vi "subVI_Mono2Go2Posv2.vi"(0 "Mono2 Motor Pos":refnum<vi>, 1 "Mono2 Wavelength (nm)":refnum<vi>, 2 "HR mode":u16(ring)=3 caption="Which HR?" items=["Excitation"=1, "Detection"=2], 3 "Postion (Unit)":dbl, 4 "ESP300 COM Port":refnum<visa-resource-name>="COM4" caption="COM Port") -> (5 "VISA resource name out":refnum<visa-resource-name>, 6 "error out":errorcluster)   [LabVIEW 2019]
panel:
  in  "Mono2 Wavelength (nm)":dbl=300.0 caption="Wavelength (nm)" min=300.0 max=1000.0 step=0.1
  in  "ESP300 Error":errorcluster
  in  "Mono2 Motor Pos":dbl caption="Motor Pos"
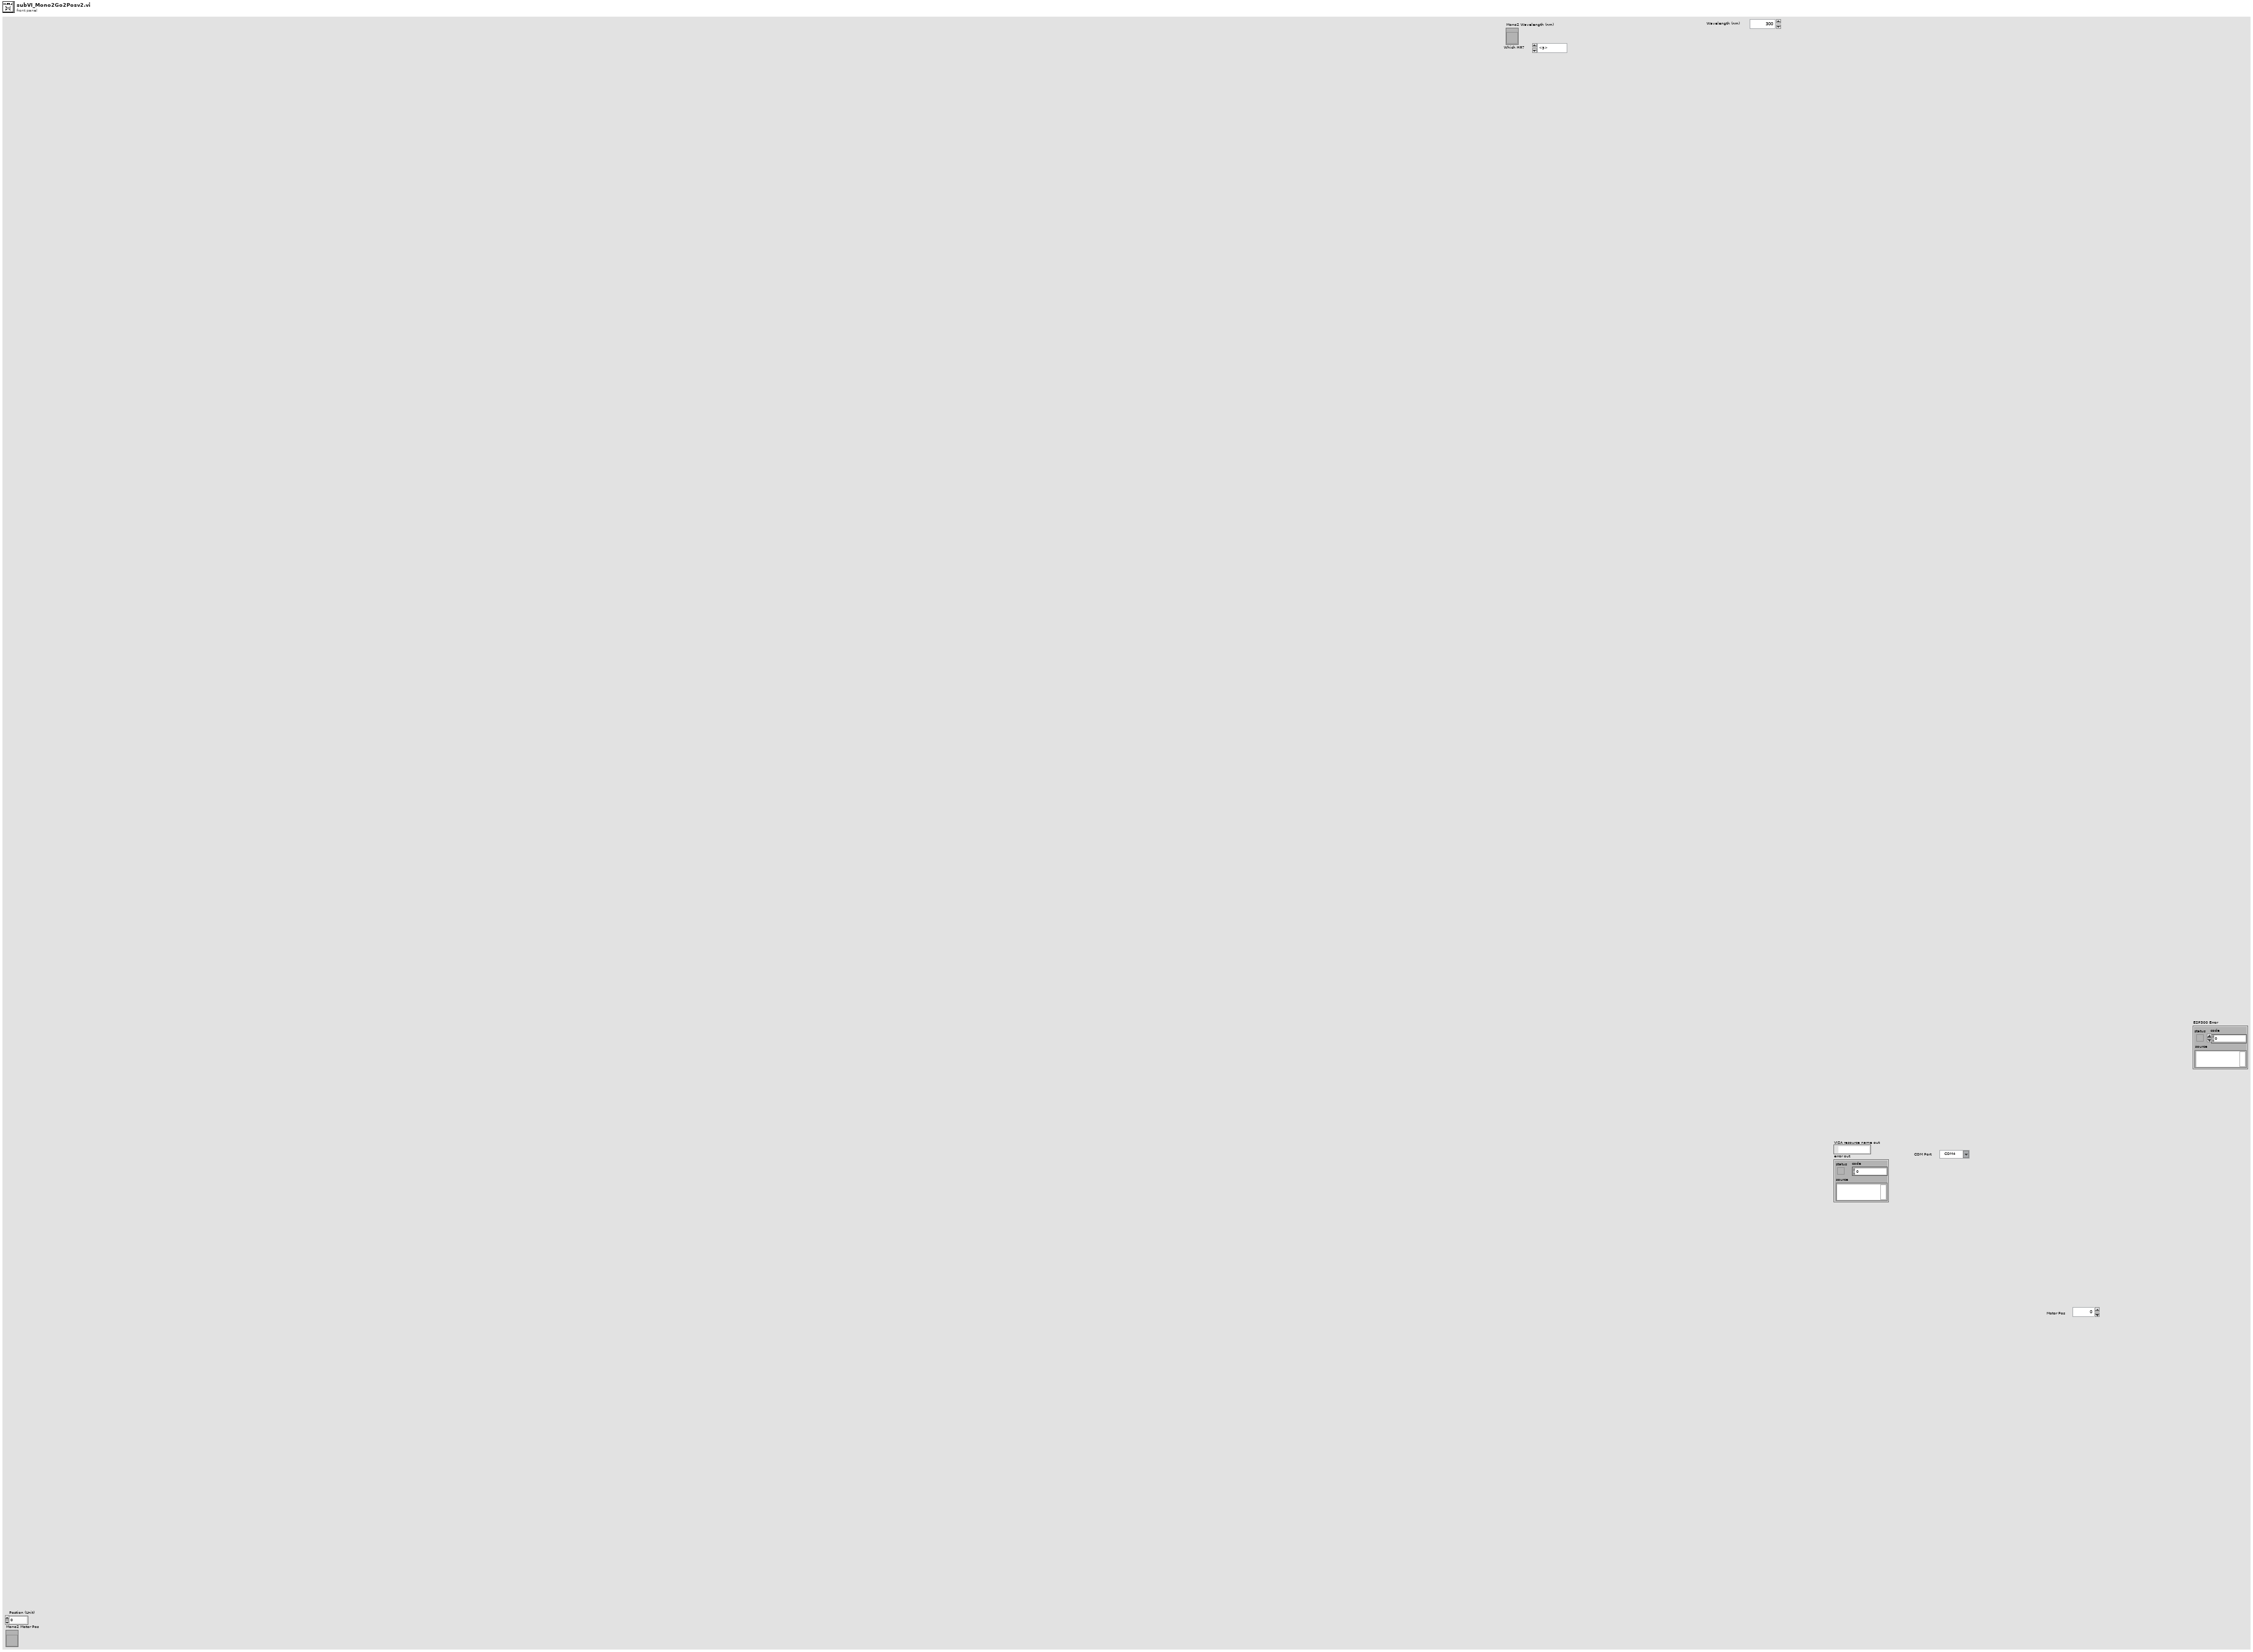
[diagram p1: front panel]
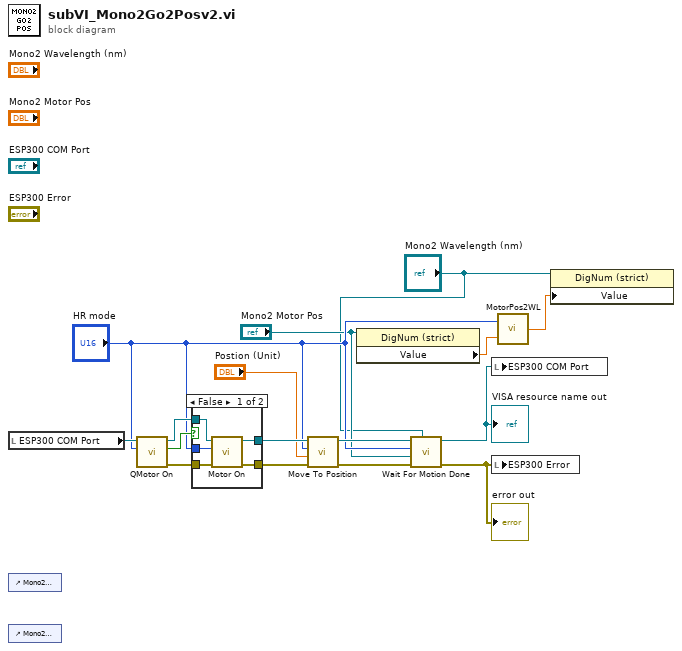
[diagram p0: block diagram]
diagram:
  n1 = local read "ESP300 COM Port"() -> (w14:refnum<visa-resource-name>)
  n2 = control-ref of="Mono2 Wavelength (nm)"() -> ()  [unwired: 1 out]
  n3 = control-ref of="Mono2 Motor Pos"() -> ()  [unwired: 1 out]
  n4 = call "QMotor On.vi"("Axis"="HR mode", "VISA resource name in"=w14) -> ("error out"=w9:errorcluster, "Motor On?"=w7:bool, "VISA resource name out"=w8:refnum<visa-resource-name>)  [unwired: 7 in]
  n5 = case shown="False" w7 {
    tunnel: "HR mode" -> [w21 _]
    tunnel: w8 -> [w20 w23]
    tunnel: w9 -> [w19 w22]
    tunnel: [w18 w23] -> w10
    tunnel: [w17 w22] -> w11
    frame False {
      n6 = call "Motor On.vi"("error in (no error)"=w19, "Axis"=w21, "VISA resource name in"=w20) -> ("error out"=w17:errorcluster, "VISA resource name out"=w18:refnum<visa-resource-name>)  [unwired: 7 in]
    }
    frame True {
    }
  }
  n7 = call "Move To Position.vi"("error in (no error)"=w11, "Postion (Unit)"="Postion (Unit)", "Axis"="HR mode", "VISA resource name in"=w10) -> ("error out"=w13:errorcluster, "VISA resource name out"=w12:refnum<visa-resource-name>)  [unwired: 6 in]
  n8 = property class="DigNum (strict)"(reference="Mono2 Motor Pos") -> ("Value"=w5:dbl)  [unwired: 1 in, 2 out]
  n9 = call "Wait For Motion Done.vi"("Mono2 Wavelength (nm)"="Mono2 Wavelength (nm)", "error in (no error)"=w13, "Mono2 Motor Pos"="Mono2 Motor Pos", "Axis"="HR mode", "VISA resource name"=w12) -> ("error out"=w16:errorcluster, "VISA resource name out"=w15:refnum<visa-resource-name>)  [unwired: 5 in]
  "VISA resource name out" <- w15
  "error out" <- w16
  n10 = local write "ESP300 COM Port"(w15) -> ()
  n11 = local write "ESP300 Error"(w16) -> ()
  n12 = call "MotorPos2WL.vi"("Mono2 Motor Position"=w5, "HR mode"="HR mode") -> ("Mono2 Center Wavelength (nm)"=w4:dbl)
  n13 = property class="DigNum (strict)"(reference="Mono2 Wavelength (nm)", "Value"=w4) -> ()  [unwired: 1 in, 2 out]
